vi "LOOP.vi"() -> ()   [LabVIEW 2018]
panel:
  out "Numeric 2":dbl
  in  "Boolean":bool
  out "Array 3":i32[](array[numeric])
  out "Numeric":dbl
  out "Array 2":i32[](array[numeric])
  out "COUNT":dbl
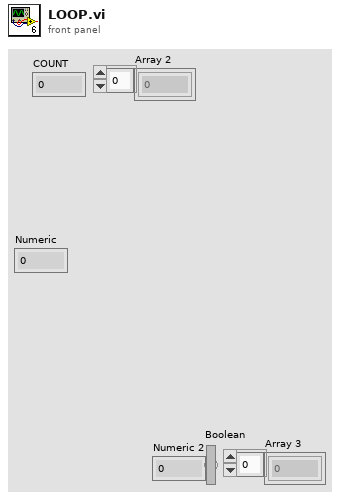
[diagram p1: front panel]
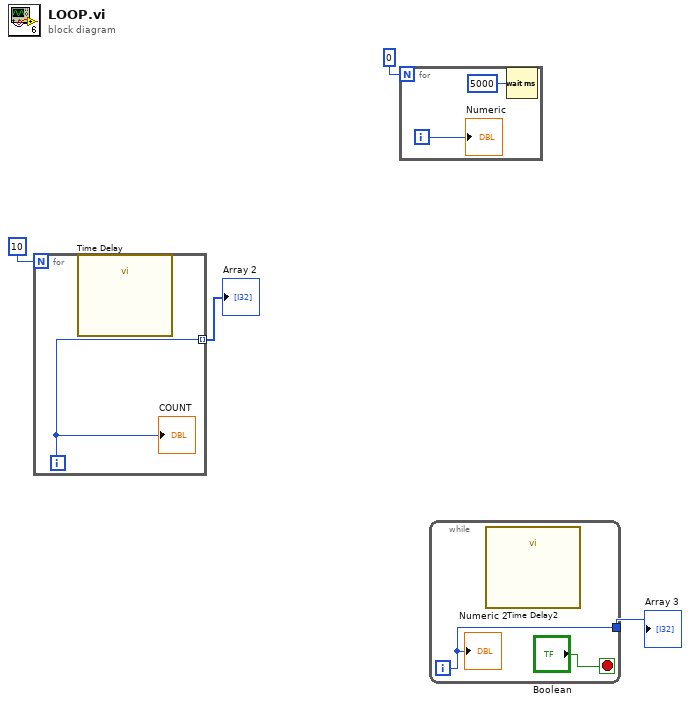
[diagram p0: block diagram]
diagram:
  n1 = for {
    N: 10 -> [_]
    tunnel: [w5] -> w3 mode=indexing
    i -> [w5]
    n2 = call "Time Delay"() -> ()  [unwired: 11 in, 1 out]
    "COUNT" <- w5
  }
  "Array 2" <- w3
  n3 = for {
    N: 0 -> [_]
    i -> [w7]
    n4 = Wait (ms)(milliseconds to wait=5000) -> ()  [unwired: 1 out]
    "Numeric" <- w7
  }
  n5 = while {
    tunnel: [w8] -> w1
    i -> [w8]
    stop <- "Boolean" stop-if-true
    n6 = call "Time Delay2"() -> ()  [unwired: 11 in, 1 out]
    "Numeric 2" <- w8
  }
  "Array 3" <- w1
